vi "force_rate_limiting.vi"(8 "Rate Limiting":bool=TRUE, 9 "Link goal":sgl[](array[numeric]), 10 "force max accel":sgl=3.0, 11 "force max vel":sgl=10.0) -> (2 "Substituted goal":sgl[](array[numeric]))   [LabVIEW 2013]
panel:
  out "Goal velocity (um/cycle)":sgl[](array[numeric])
  # "Locals:"
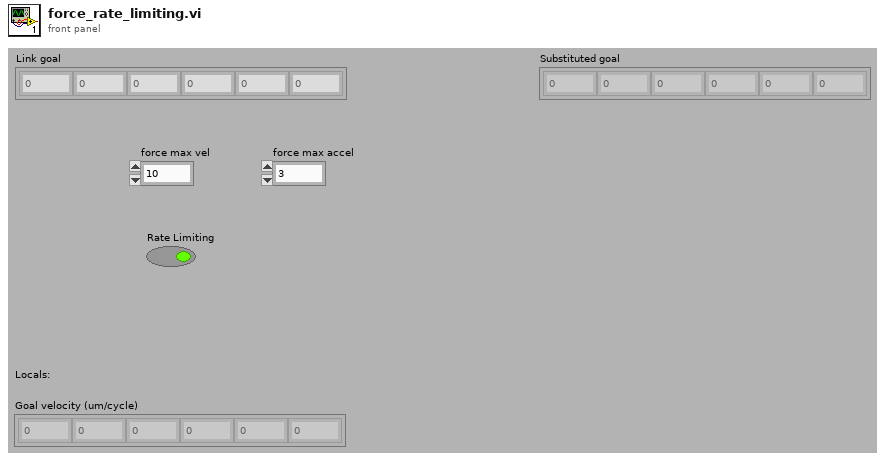
[diagram p1: front panel]
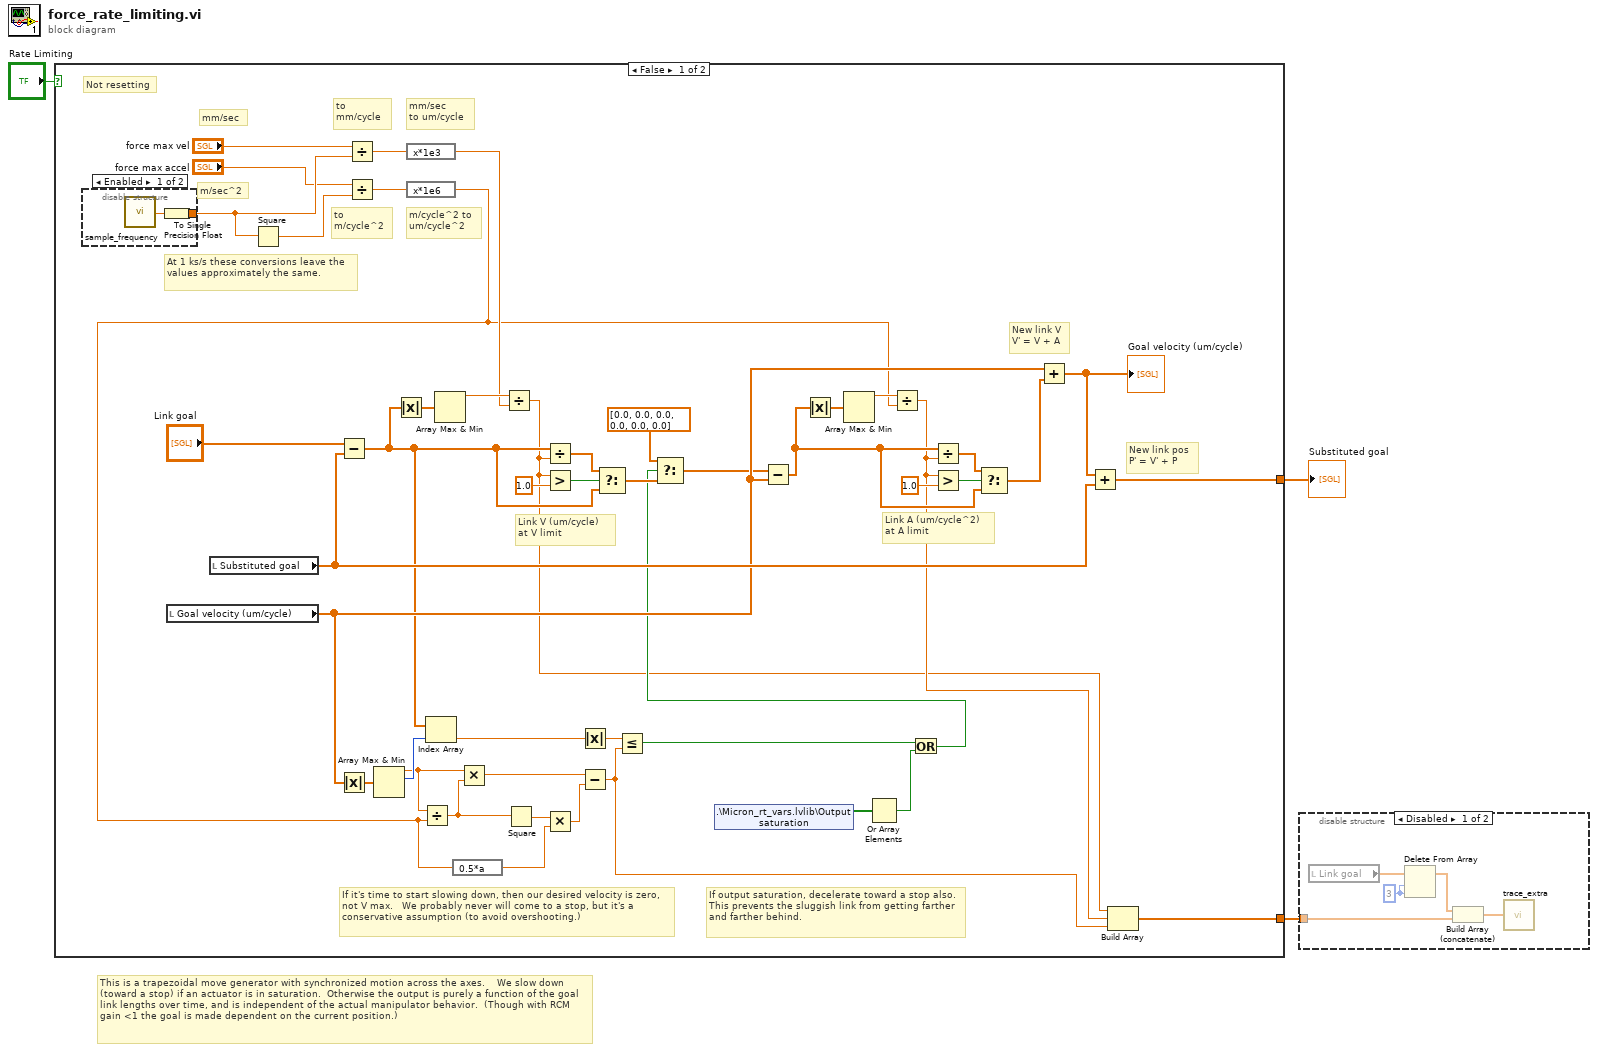
[diagram p0: block diagram]
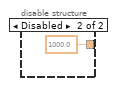
[diagram p3: hidden frame]
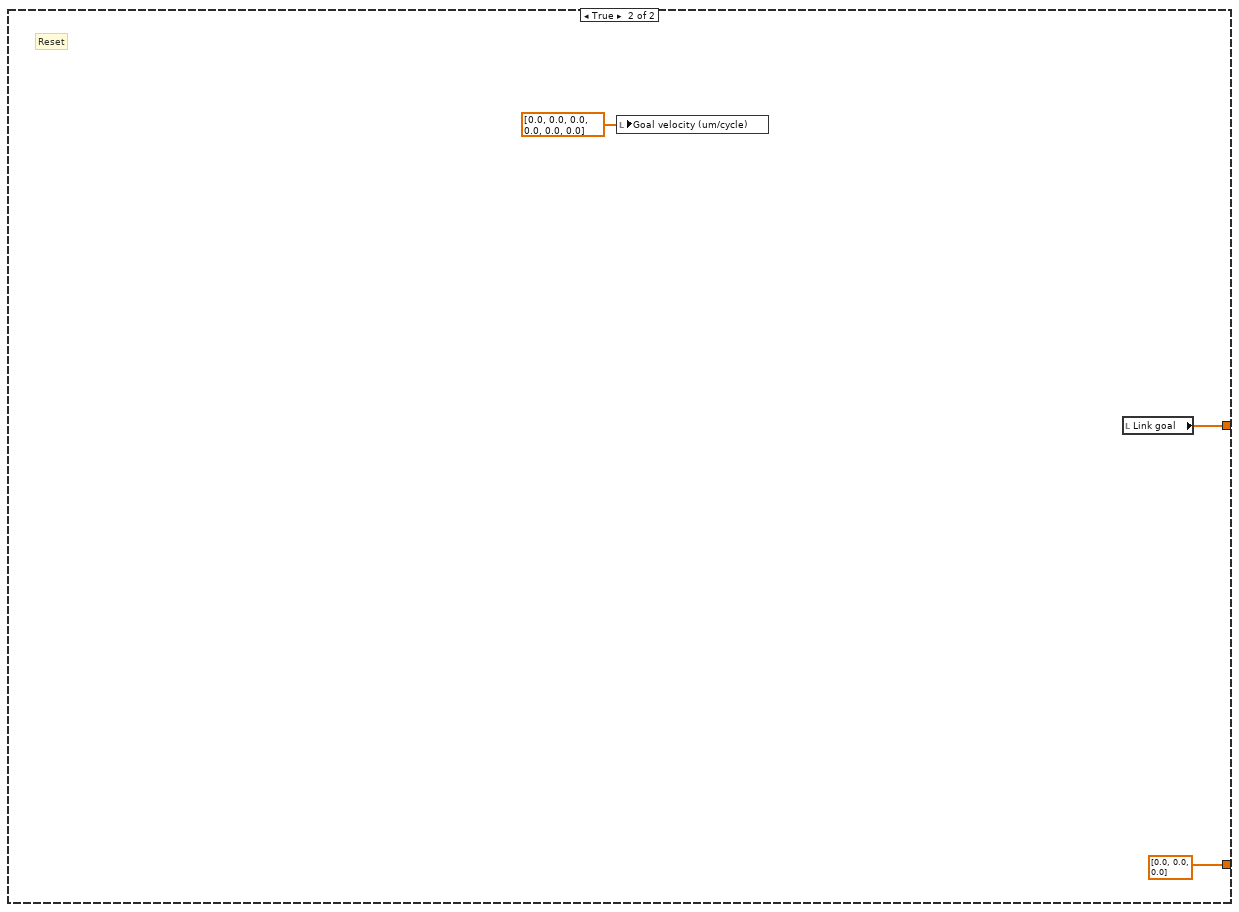
[diagram p4: hidden frame]
diagram:
  # "This is a trapezoidal move generator with synchronized motion across the axes.    We slow down (toward a stop) if an actuator is in saturation.  Otherwise the output is purely a function of the goal link lengths over time, and is independent of the actual manipulator behavior.  (Though with RCM gain <1 the goal is made dependent on the current position.)"
  n1 = case shown="False" "Rate Limiting" {
    tunnel: [w38 w54] -> w3
    tunnel: [w30 sgl[] [0.0, 0.0, 0.0]] -> w2
    frame False {
      # "If output saturation, decelerate toward a stop also.  This prevents the sluggish link from getting farther and farther behind."
      # "If it's time to start slowing down, then our desired velocity is zero, not V max.   We probably never will come to a stop, but it's a conservative assumption (to avoid overshooting.)"
      # "New link pos\nP' = V' + P"
      # "New link V\nV' = V + A"
      # "Link A (um/cycle^2)\nat A limit"
      # "Link V (um/cycle) \nat V limit"
      # "Not resetting"
      # "At 1 ks/s these conversions leave the values approximately the same."
      # "to \nm/cycle^2"
      # "m/sec^2"
      # "mm/sec"
      # "to\nmm/cycle"
      # "m/cycle^2 to\num/cycle^2"
      # "mm/sec \nto um/cycle"
      n2 = disable-structure shown="Enabled" {
        disable-tunnel: [w51 sgl 1000.0] -> w44
        frame Enabled {
          n3 = call "sample_frequency.vi"() -> ("Sample frequency"=w52:dbl)
          n4 = To Single Precision Float(number=w52) -> (single precision float=w51:sgl)
        }
        frame Disabled {
        }
      }
      n5 = local read "Goal velocity (um/cycle)"() -> (w22:sgl[])
      n6 = local read "Substituted goal"() -> (w39:sgl[])
      n7 = Square(x=w44) -> (x^2=w45:sgl)
      n8 = Subtract(x="Link goal", y=w39) -> (x-y=w20:sgl[])
      n9 = Absolute Value(x=w22) -> (abs(x)=w29:sgl[])
      n10 = Divide(x="force max vel", y=w44) -> (x/y=w49:sgl)
      n11 = Divide(x="force max accel", y=w45) -> (x/y=w46:sgl)
      n12 = Array Max & Min(array=w29) -> (max value=w28:sgl, max index (indices)=w50:i32)  [unwired: 2 out]
      n13 = Absolute Value(x=w20) -> (abs(x)=w48:sgl[])
      n14 = expression code="x*1e3"(w49) -> (w43:sgl)
      n15 = expression code="x*1e6"(w46) -> (w21:sgl)
      n16 = Divide(x=w28, y=w21) -> (x/y=w27:sgl)
      n17 = Index Array(array=w20, index=w50) -> (element=w7:sgl)
      n18 = Array Max & Min(array=w48) -> (max value=w47:sgl)  [unwired: 3 out]
      n19 = expression code="0.5*a"(w21) -> (w25:sgl)
      n20 = Multiply(x=w28, y=w27) -> (x*y=w24:sgl)
      n21 = Divide(x=w47, y=w43) -> (x/y=w8:sgl)
      n22 = Square(x=w27) -> (x^2=w26:sgl)
      n23 = Divide(x=w20, y=w8) -> (x/y=w41:sgl[])
      n24 = Greater?(x=w8, y=sgl 1.0) -> (0:w10:bool)
      n25 = Multiply(x=w26, y=w25) -> (x*y=w23:sgl)
      n26 = Absolute Value(x=w7) -> (abs(x)=w6:sgl)
      n27 = Subtract(x=w24, y=w23) -> (x-y=w16:sgl)
      n28 = Select(t=w41, s=w10, f=w20) -> (s? t:f=w19:sgl[])
      n29 = Less Or Equal?(x=w6, y=w16) -> (x <= y?=w14:bool)
      n30 = shared-variable ".\\Micron_rt_vars.lvlib\\Output saturation"() -> (w15:bool[])  [unwired: 1 in, 1 out]
      n31 = Or Array Elements(Boolean array=w15) -> (logical OR=w12:bool)
      n32 = Or(x=w14, y=w12) -> (x .or. y?=w13:bool)
      n33 = Select(t=sgl[] [0.0, 0.0, 0.0, 0.0, 0.0, 0.0] ("Goal velocity (um/cycle)"), s=w13, f=w19) -> (s? t:f=w17:sgl[])
      n34 = Subtract(x=w17, y=w22) -> (x-y=w31:sgl[])
      n35 = Absolute Value(x=w31) -> (abs(x)=w37:sgl[])
      n36 = Array Max & Min(array=w37) -> (max value=w36:sgl)  [unwired: 3 out]
      n37 = Divide(x=w36, y=w21) -> (x/y=w9:sgl)
      n38 = Divide(x=w31, y=w9) -> (x/y=w34:sgl[])
      n39 = Greater?(x=w9, y=sgl 1.0) -> (0:w11:bool)
      n40 = Select(t=w34, s=w11, f=w31) -> (s? t:f=w33:sgl[])
      n41 = Add(x=w22, y=w33) -> (x+y=w32:sgl[])
      "Goal velocity (um/cycle)" <- w32
      n42 = Add(x=w32, y=w39) -> (x+y=w38:sgl[])
      n43 = Build Array(w8, w9, w16) -> (w30:sgl[])
    }
    frame True {
      # "Reset"
      n44 = local write "Goal velocity (um/cycle)"(sgl[] [0.0, 0.0, 0.0, 0.0, 0.0, 0.0] ("Goal velocity (um/cycle)")) -> ()
      n45 = local read "Link goal"() -> (w54:sgl[])
    }
  }
  "Substituted goal" <- w3
  n46 = disable-structure shown="Disabled" {
    disable-tunnel: w2 -> [w57 _]
    frame Disabled {
      w60 = 3 ("index")
      n47 = local read "Link goal"() -> (w61:sgl[])
      n48 = Delete From Array(array=w61, length=w60, index=w60) -> (array with subset deleted=w59:sgl[])  [unwired: 1 out]
      n49 = Build Array (concatenate)(w59, w57) -> (w58:sgl[])
      n50 = call "trace_extra.vi"("Extra trace data"=w58) -> ()  [unwired: 1 in]
    }
    frame Enabled {
    }
  }
